vi "Feature Toggle Page.vi"(5 "feature disabled vi":string, 7 "feature enabled vi":string, 8 "error in (no error)":errorcluster, 9 "Node Ptr":T1 format="%.0x", 10 "feature name":string, 11 "SubPanel in":refnum<vi>) -> (0 "error out":errorcluster)   [LabVIEW 2015, in "Engine Simulation Toolkit System Explorer.lvlib"]
uses:
  Engine Simulation Toolkit System Explorer.lvlib
  <vilib>/NI Veristand/Custom Device API/Custom Device Item Ref.ctl
  <vilib>/NI Veristand/Custom Device API/Custom Device API.lvlib
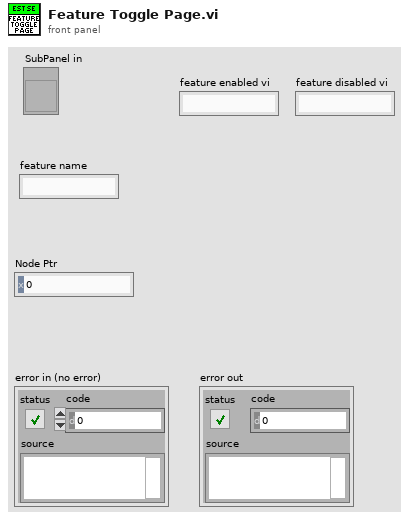
[diagram p1: front panel]
types:
  T1 = typedef "Custom Device API.lvlib/Custom Device Item Ref.ctl" = u64
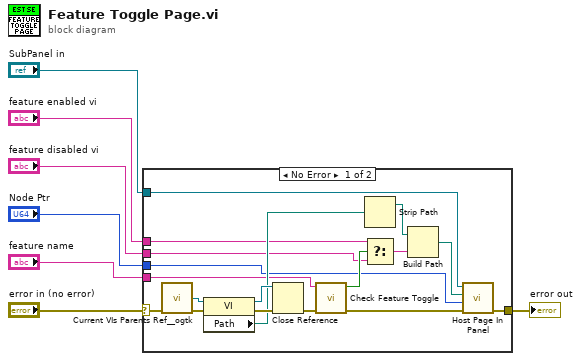
[diagram p0: block diagram]
diagram:
  n1 = case shown="No Error" "error in (no error)" {
    selector: "error in (no error)" -> [w24 w25]
    tunnel: [w18 w25] -> w6
    tunnel: "feature disabled vi" -> [w13 _]
    tunnel: "feature enabled vi" -> [w12 _]
    tunnel: "SubPanel in" -> [w11 _]
    tunnel: "Node Ptr" -> [w9 _]
    tunnel: "feature name" -> [w8 _]
    frame No Error {
      n2 = call <userlib>:"Current VIs Parents Ref__ogtk.vi"() -> ("Calling VI's Reference"=w19:refnum<vi>)  [unwired: 2 in]
      n3 = property class="VI"(reference=w19, error in=w24) -> (reference out=w21:refnum<vi>, error out=w22:errorcluster, "Path"=w20:path)
      n4 = Close Reference(reference=w21, error in (no error)=w22) -> (error out=w23:errorcluster)
      n5 = call "Check Feature Toggle.vi"("error in (no error)"=w23, "feature name"=w8) -> ("error out"=w10:errorcluster, "feature enabled"=w14:bool)  [unwired: 8 in]
      n6 = Strip Path(path=w20) -> (stripped path=w15:path)  [unwired: 1 out]
      n7 = Select(t=w12, s=w14, f=w13) -> (s? t:f=w16:string)
      n8 = Build Path(base path=w15, name or relative path=w16) -> (appended path=w17:path)
      n9 = call "Host Page In Panel.vi"("error in (no error)"=w10, "Node Ptr"=w9, "vi path"=w17, "SubPanel in"=w11) -> ("error out"=w18:errorcluster)  [unwired: 7 in]
    }
    frame Error {
    }
  }
  "error out" <- w6
